vi "Load Reference.vi"(8 "error in (no error)":errorcluster, 10 "Reference":refnum<vi>, 11 "ActiveX Control in":refnum<class "ActiveXContainer.lvclass">) -> (0 "error out":errorcluster, 3 "ActiveX Control out":refnum<class "ActiveXContainer.lvclass">)   [LabVIEW 2020, in "WebView2 QControl.lvlib" / "ActiveXContainer.lvclass"]
doc: "The <b>Load Reference VI</b> is a dynamic dispatch VI that must be overwritten in every QControl Class and must <b>Call Parent Method</b>. This recursively loads the reference of the control to the data space for the Control Class up the inheritance hierarchy (class hierarchy). These references must be loaded in this way to use all of the built-in properties.\n\nThe reference input is the reference type needed for the control but is coerced to Generic. It should be cast back to the correct type before bundling into the class private data. The pre-casted \"Generic\" reference is wired as input to the <b>Call Parent Method</b>.\n<b> </b> <b> </b>\n©2016 Q Software Innovations, LLC (QSI)\nwritten by Quentin Alldredge\nproduced in LabVIEW 2015\n\nsupport@qsoftwareinnovations.com\nwww.qsoftwareinnovations.com\n\nAll rights reserved.\n\nRedistribution and use in source and binary forms, with or without modification, are permitted provided that the following conditions are met:\n\n * Redistributions of source code must retain the above copyright notice, this list of conditions and the following disclaimer.\n * Redistributions in binary form must reproduce the above copyright notice, this list of conditions and the following disclaimer in the documentation and/or other materials provided with the distribution.\n * Neither the name of Q Software Innovations, LLC. nor the names of its contributors may be used to endorse or promote products derived from this software without specific prior written permission.\n\nTHIS SOFTWARE IS PROVIDED BY THE COPYRIGHT HOLDERS AND CONTRIBUTORS \"AS IS\" AND ANY EXPRESS OR IMPLIED WARRANTIES, INCLUDING, BUT NOT LIMITED TO, THE IMPLIED WARRANTIES OF MERCHANTABILITY AND FITNESS FOR A PARTICULAR PURPOSE ARE DISCLAIMED. IN NO EVENT SHALL THE COPYRIGHT OWNER OR CONTRIBUTORS BE LIABLE FOR ANY DIRECT, INDIRECT, INCIDENTAL, SPECIAL, EXEMPLARY, OR CONSEQUENTIAL DAMAGES (INCLUDING, BUT NOT LIMITED TO, PROCUREMENT OF SUBSTITUTE GOODS OR SERVICES; LOSS OF USE, DATA, OR PROFITS; OR BUSINESS INTERRUPTION) HOWEVER CAUSED AND ON ANY THEORY OF LIABILITY, WHETHER IN CONTRACT, STRICT LIABILITY, OR TORT (INCLUDING NEGLIGENCE OR OTHERWISE) ARISING IN ANY WAY OUT OF THE USE OF THIS SOFTWARE, EVEN IF ADVISED OF THE POSSIBILITY OF SUCH DAMAGE."
uses:
  ActiveXContainer.lvclass
  ActiveXContainer.lvclass/ActiveXContainer.ctl
  <vilib>/QSI/QControls/QControl Classes/Control/Control.lvclass
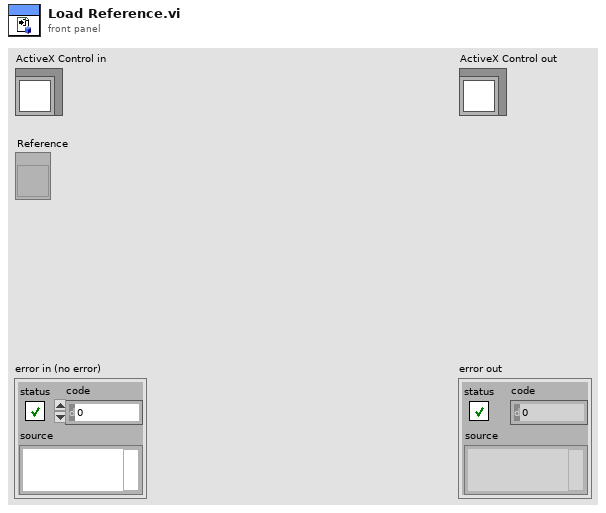
[diagram p1: front panel]
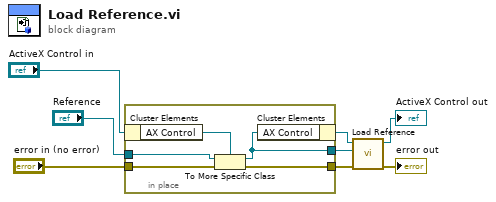
[diagram p0: block diagram]
diagram:
  n1 = in-place {
    in-place-border: "Reference" -> [w13]
    in-place-border: "error in (no error)" -> [w12]
    in-place-border: [w9] -> w2
    in-place-border: [w11] -> w1
    n2 = in-place-cluster #1("ActiveX Control in") -> ("AX Control"=w10:refnum<vi>)
    n3 = To More Specific Class(target class=w10, reference=w13, error in=w12) -> (specific class reference=w9:refnum<vi>, error out=w11:errorcluster)
    n4 = in-place-cluster #1("AX Control"=w9) -> (w5:refnum<class "ActiveXContainer.lvclass">)
  }
  n5 = call-parent "Load Reference.vi"("error in (no error)"=w1, "Reference"=w2, "Control in"=w5) -> ("error out"=→"error out":errorcluster, "Control out"=→"ActiveX Control out":refnum<class "ActiveXContainer.lvclass">)  [unwired: 7 in]
